vi "MB Serial Transmit.vi"(7 "Serial Parameters":T1 {"Slave Address" format="%.0x"}, 8 "error in (no error)":errorcluster, 10 "Modbus Data Unit":T2={"Function Code"=1, "Data"=[]} {"Function Code" items=["Read Coils"=1, "Read Discrete Inputs"=2, "Read Holding Registers"=3, "Read Input Registers"=4, "Write Single Coil"=5, "Write Single Register"=6, "Read Exception Status"=7, "Write Multiple Coils"=15, "Write Multiple Registers"=16]; "Data" format="%.0x"}, 11 "VISA resource name":refnum<visa-resource-name>) -> (0 "error out":errorcluster, 3 "VISA resource name out":refnum<visa-resource-name>)   [LabVIEW 2012]
uses:
  MB Modbus Data Unit.ctl
panel:
  # "VI Name: MB Serial Transmit.vi\nPurpose: Sends a Modbus message.\nReentrant."
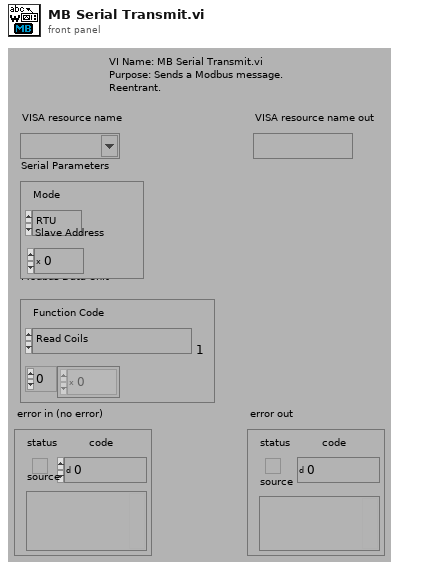
[diagram p1: front panel]
types:
  T1 = cluster{"Mode":enum16{"RTU", "ASCII"}, "Slave Address":u8}
  T2 = typedef "MB Modbus Data Unit.ctl" = cluster{"Function Code":u8, "Data":u8[]}
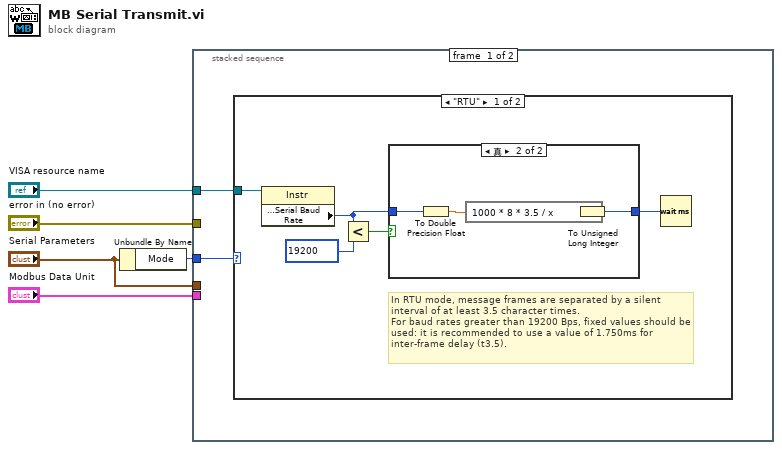
[diagram p0: block diagram]
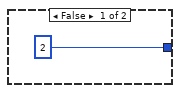
[diagram p2: hidden frame]
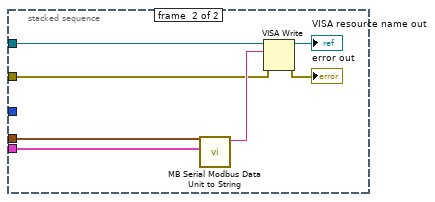
[diagram p4: hidden frame]
diagram:
  n1 = Unbundle By Name("Serial Parameters") -> ("Mode"=w2:enum16{"RTU", "ASCII"})
  n2 = stacked-sequence {
    tunnel: w2 -> [w6 _]
    tunnel: "Modbus Data Unit" -> [_ w19]
    tunnel: "VISA resource name" -> [w7 w21]
    tunnel: "error in (no error)" -> [_ w20]
    tunnel: "Serial Parameters" -> [_ w18]
    frame #0 {
      n3 = case shown="\"RTU\"" w6 {
        tunnel: w7 -> [w12 _]
        frame "RTU" {
          # "In RTU mode, message frames are separated by a silent interval of at least 3.5 character times.\nFor baud rates greater than 19200 Bps, fixed values should be used: it is recommended to use a value of 1.750ms for inter-frame delay (t3.5)."
          n4 = property class="Instr"(reference=w12) -> ("Serial Settings:Serial Baud Rate"=w10:u32)  [unwired: 1 in, 2 out]
          n5 = Less?(x=w10, y=u32 19200 ("Serial Settings:Serial Baud Rate")) -> (x < y?=w8:bool)
          n6 = case shown="真" w8 {
            tunnel: [u32 2 w15] -> w11
            tunnel: w10 -> [_ w14]
            frame False {
            }
            frame True {
              n7 = To Double Precision Float(number=w14) -> (double precision float=w17:dbl)
              n8 = expression code="1000 * 8 * 3.5 / x"(w17) -> (w16:dbl)
              n9 = To Unsigned Long Integer(number=w16) -> (unsigned 32bit integer=w15:u32)
            }
          }
          n10 = Wait (ms)(milliseconds to wait=w11) -> ()  [unwired: 1 out]
        }
        frame "ASCII" {
        }
      }
    }
    frame #1 {
      n11 = call "MB Serial Modbus Data Unit to String.vi"("Modbus Data Unit"=w19, "Serial Parameters"=w18) -> ("String"=w24:string)  [unwired: 3 in, 6 out]
      n12 = VISA Write(VISA resource name=w21, write buffer=w24, error in (no error)=w20) -> (VISA resource name out=→"VISA resource name out":refnum<visa-resource-name>, error out=→"error out":errorcluster)  [unwired: 1 out]
    }
  }
